vi "Temperature Sensing Test_v2.vi"(8 "error in (no error)":errorcluster, 11 "ContolBoard VISA":refnum<visa-resource-name>="ControlBoard") -> (0 "error out":errorcluster, 2 "Rel. Humidity":dbl, 3 "Temperature":dbl)   [LabVIEW 2022 SP3]
uses:
  <vilib>/Instr/_visa.llb/VISA Flush IO Buffer Mask.ctl
panel:
  out "Actual Result":string
  out "VISA resource OUT":refnum<visa-resource-name>
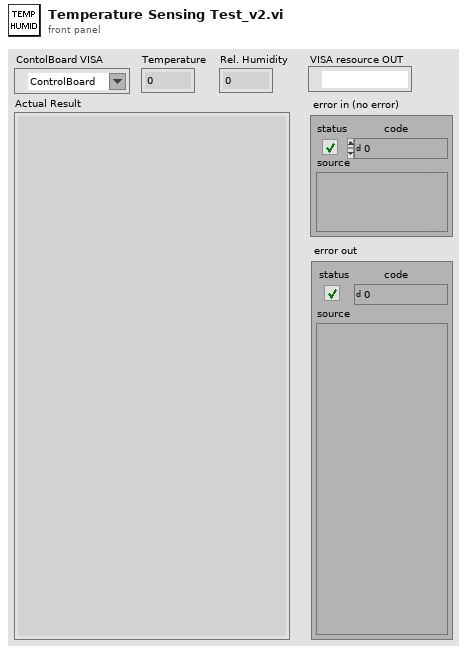
[diagram p1: front panel]
types:
  T1 = typedef "VISA Flush IO Buffer Mask.ctl" = u16
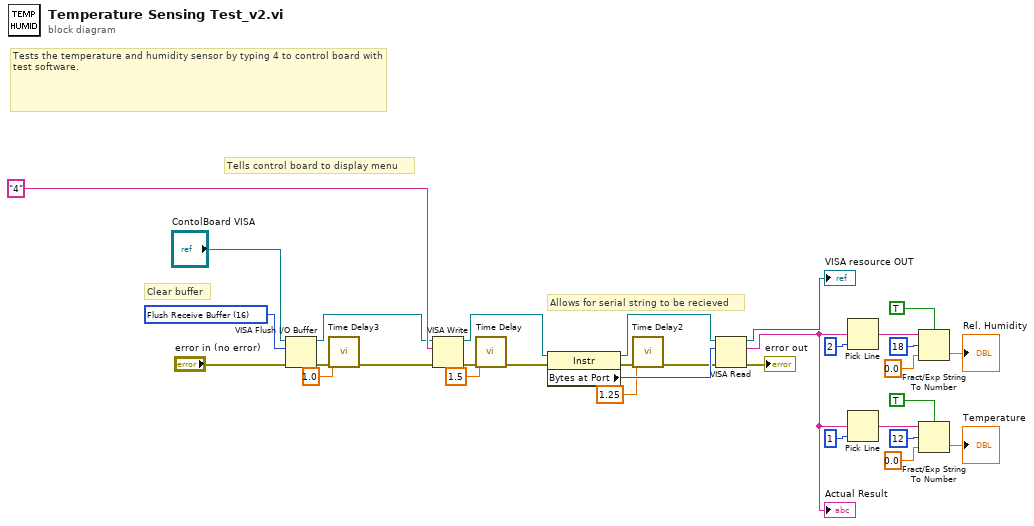
[diagram p0: block diagram]
diagram:
  w29 = T1 16 items=["Flush Receive Buffer"=16, "Write Transmit Buffer to Device"=32, "Flush Receive Buffer (No I/O)"=64, "Flush Transmit Buffer"=128] ("Mask")
  # "Tests the temperature and humidity sensor by typing 4 to control board with test software."
  # "Clear buffer"
  # "Allows for serial string to be recieved"
  # "Tells control board to display menu"
  n1 = VISA Flush I/O Buffer(VISA resource name="ContolBoard VISA", mask (16)=w29, error in (no error)="error in (no error)") -> (VISA resource name out=w27:refnum<visa-resource-name>, error out=w5:errorcluster)
  n2 = call "Time Delay3"("error in (no error)"=w5, "Delay Time (s)"=1.0) -> ("error out"=w4:errorcluster)  [unwired: 9 in]
  n3 = VISA Write(VISA resource name=w27, write buffer="4", error in (no error)=w4) -> (VISA resource name out=w25:refnum<visa-resource-name>, error out=w28:errorcluster)  [unwired: 1 out]
  n4 = call "Time Delay"("error in (no error)"=w28, "Delay Time (s)"=1.5) -> ("error out"=w26:errorcluster)  [unwired: 9 in]
  n5 = property class="Instr"(reference=w25, error in=w26) -> (reference out=w31:refnum<visa-resource-name>, error out=w20:errorcluster, "Bytes at Port"=w30:u32)
  n6 = call "Time Delay2"("error in (no error)"=w20, "Delay Time (s)"=1.25) -> ("error out"=w19:errorcluster)  [unwired: 9 in]
  n7 = VISA Read(VISA resource name=w31, byte count=w30, error in (no error)=w19) -> (VISA resource name out=→"VISA resource OUT":refnum<visa-resource-name>, read buffer=w8:string, error out=→"error out":errorcluster)  [unwired: 1 out]
  "Actual Result" <- w8
  n8 = Pick Line(multi-line string=w8, line index=2) -> (output string=w12:string)  [unwired: 1 in]
  n9 = Pick Line(multi-line string=w8, line index=1) -> (output string=w17:string)  [unwired: 1 in]
  n10 = Fract/Exp String To Number(use system decimal point (T)=TRUE, string=w12, offset=18, default (0 dbl)=0.0 ("default (0 DBL)")) -> (number=→"Rel. Humidity":dbl)  [unwired: 1 out]
  n11 = Fract/Exp String To Number(use system decimal point (T)=TRUE, string=w17, offset=12, default (0 dbl)=0.0 ("default (0 DBL)")) -> (number=→"Temperature":dbl)  [unwired: 1 out]
